vi "PRIME Detector Send START.vi"(5 "Observation":T1={"Priority"=0, "ID"="", "Observer"="", "Obj Name"="", "Obj Type"="", "RA and DEC String"={"RA"="HH:MM:SS.nnn", "DEC"="DEG:arcmin:arcsec.nn"}, "Filter Wheel 1"="", "Filter Wheel 2"="", "Integration Time"=0.0, "Observation Status"=enum."Error", "Offsets"={"RA"=0.0, "DEC"=0.0, "ROT"=0.0}, "Images"=0, "Dither Options"={"Dither"=enum."None", "Dither Radius"=0.0, "Dither Points"=0, "Dither Phase"=0.0}, "Comment 1"="", "Comment 2"=""}, 7 "Detector Config":T6={"Detector"=0, "Offsets"=[[0, 0, 0, 0, 0, 0, 0, 0, 0, 0, 0, 0, 0, 0, 0, 0, 0, 0, 0, 0, 0, 0, 0, 0, 0, 0, 0, 0, 0, 0, 0, 0]], "Detector Computer"={"Machine"="192.168.121.11", "Password"="rSL!nux23456", "FITS File Path"="", "Port"=44444, "Header Path"="", "Name"=""}, "FITS hdr template0"=path "", "FITS hdr template1"=path "", "FITS Data File Path"=path "", "FITS Detector Settings"={"Exp Time Short"=0.0, "# of Frames"=0.0, "Exp Time Long"=0.0, "# of Groups"=0.0, "Object Name"="", "Object"="", "Obs Type"="", "Image Type"="", "Observer"="", "Observer Affiliation"=""}, "Sim Folder"=path "", "Integration Mode"=enum."SSR", "Integration Time"=0.0, "Frame Int Time"=0.0} {"Offsets" format="%04x"; "Detector" items=["0", "1", "2"]}, 8 "error in (no error)":errorcluster, 9 "timeout (120s)":dbl=120.0, 10 "Exposure Time":dbl, 11 "connection ID":refnum<k5>[](array[refnum])) -> (0 "error out":errorcluster, 1 "Image Map":map{string, T10}(c390), 2 "Status out":T11, 3 "connection ID out":refnum<k5>[](array[refnum]))   [LabVIEW 2024, in "PRIME Detector.lvclass"]
uses:
  PRIME Detector.lvclass
  PRIME Detector cluster Status.ctl
  Detector Image typedef cluster.ctl
  RIMAS Detector Config.ctl
  RIMAS Detector Server Config.ctl
  RIMAS Observation Config.ctl
  Detector enum Detector Integration Mode.ctl
  typedefs/CC cluster Observation.ctl
  Observation Queue/CC enum Observation Status.ctl
  Telescope/CC cluster Telescope Offsets.ctl
  typedefs/CC cluster Observation Dither Options.ctl
  typedefs/CC enum Dither Selection.ctl
  3c100308-56f2-4219-aefe-58094781b1bc.vi
  Detector Class.lvclass
panel:
  out "Status":string
  out "Responses":string[](array[string])
  # "sec"
  # "sec"
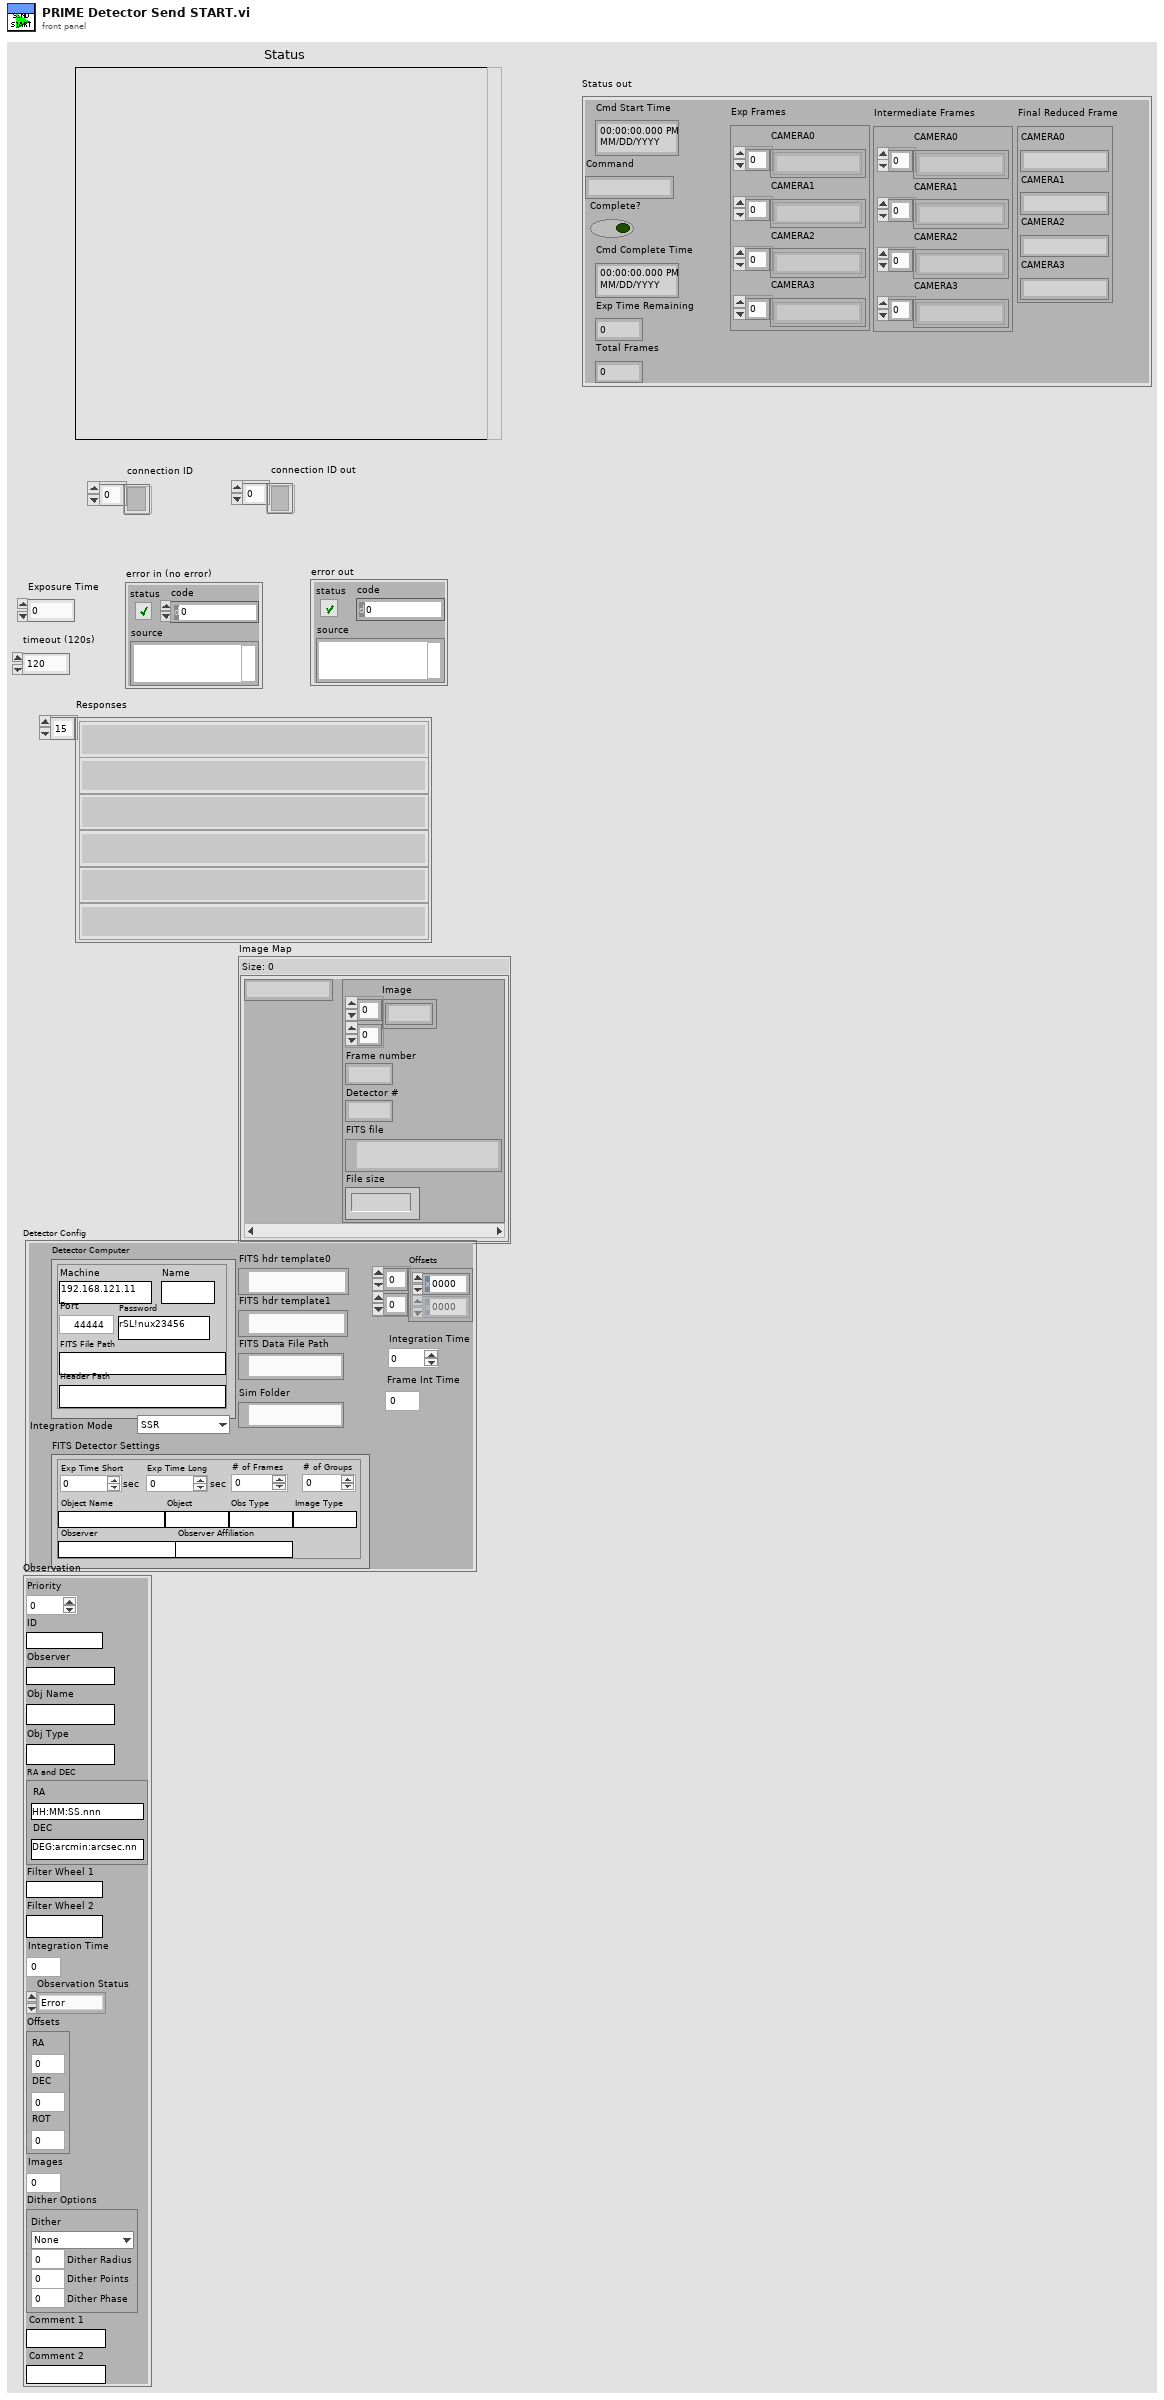
[diagram p1: front panel]
types:
  T1 = typedef "CC cluster Observation.ctl" = cluster{"Priority":i32, "ID":string, "Observer":string, "Obj Name":string, "Obj Type":string, "RA and DEC String":cluster{"RA":string, "DEC":string}, "Filter Wheel 1":string, "Filter Wheel 2":string, "Integration Time":dbl, "Observation Status":T2, "Offsets":T3, "Images":i32, "Dither Options":T4, "Comment 1":string, "Comment 2":string}
  T2 = typedef "CC enum Observation Status.ctl" = enum16{"Ready", "Running", "Done", "Error"}
  T3 = typedef "CC cluster Telescope Offsets.ctl" = cluster{"RA":dbl, "DEC":dbl, "ROT":dbl}
  T4 = typedef "CC cluster Observation Dither Options.ctl" = cluster{"Dither":T5, "Dither Radius":dbl, "Dither Points":i32, "Dither Phase":dbl}
  T5 = typedef "CC enum Dither Selection.ctl" = enum16{"None", "Circle", "Random"}
  T6 = typedef "RIMAS Detector Config.ctl" = cluster{"Detector":u16, "Offsets":u16[][], "Detector Computer":T7, "FITS hdr template0":path, "FITS hdr template1":path, "FITS Data File Path":path, "FITS Detector Settings":T8, "Sim Folder":path, "Integration Mode":T9, "Integration Time":dbl, "Frame Int Time":dbl}
  T7 = typedef "RIMAS Detector Server Config.ctl" = cluster{"Machine":string, "Password":string, "FITS File Path":string, "Port":u16, "Header Path":string, "Name":string}
  T8 = typedef "RIMAS Observation Config.ctl" = cluster{"Exp Time Short":dbl, "# of Frames":dbl, "Exp Time Long":dbl, "# of Groups":dbl, "Object Name":string, "Object":string, "Obs Type":string, "Image Type":string, "Observer":string, "Observer Affiliation":string}
  T9 = typedef "Detector enum Detector Integration Mode.ctl" = enum16{"SSR", "CDS", "MEAN", "MEDIAN", "MODE", "MIIN", "MAX"}
  T10 = typedef "Detector Class.lvclass/Detector Image typedef cluster.ctl" = cluster{"Image":sgl[][], "Frame number":i32, "Detector #":u16, "FITS file":path, "File size":i64}
  T11 = typedef "PRIME Detector cluster Status.ctl" = cluster{"Cmd Start Time":timestamp, "Command":string, "Complete?":bool, "Cmd Complete Time":timestamp, "Exp Time Remaining":dbl, "Total Frames":i32, "Exp Frames":cluster{"CAMERA0":string[], "CAMERA1":string[], "CAMERA2":string[], "CAMERA3":string[]}, "Intermediate Frames":cluster{"CAMERA0":string[], "CAMERA1":string[], "CAMERA2":string[], "CAMERA3":string[]}, "Final Reduced Frame":cluster{"CAMERA0":string, "CAMERA1":string, "CAMERA2":string, "CAMERA3":string}}
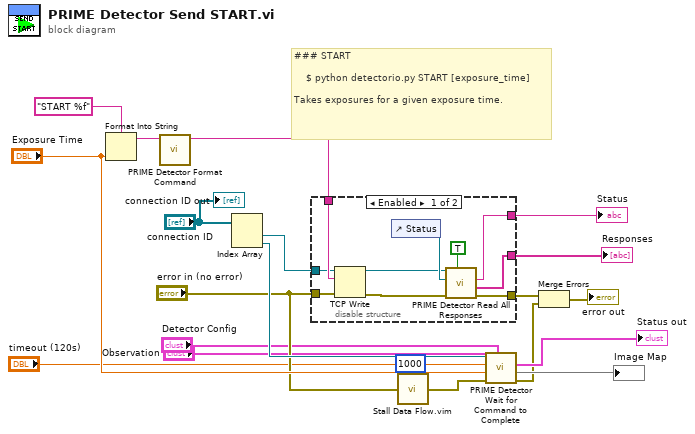
[diagram p0: block diagram]
diagram:
  # "### START\n\n    $ python detectorio.py START [exposure_time]\n\nTakes exposures for a given exposure time."
  n1 = Format Into String(format string="START %f" ("Command"), "Exposure Time") -> (resulting string=w14:string)  [unwired: 2 in, 1 out]
  n2 = call "PRIME Detector Format Command.vi"("Command"=w14) -> ("TCP String"=w20:string)  [unwired: 10 in]
  n3 = Index Array(array="connection ID") -> (element #1=w16:refnum<k5>, element #2=w13:refnum<k5>)  [unwired: 2 in]
  n4 = disable-structure shown="Enabled" {
    disable-tunnel: w20 -> [w30 _]
    disable-tunnel: "error in (no error)" -> [w29 _]
    disable-tunnel: [w28 _] -> w19
    disable-tunnel: [w27 _] -> w17
    disable-tunnel: w16 -> [w25 _]
    disable-tunnel: [w23 _] -> w15
    frame Enabled {
      n5 = TCP Write(connection ID=w25, data in=w30, error in (no error)=w29) -> (connection ID out=w24:refnum<k5>, error out=w21:errorcluster)  [unwired: 1 in, 1 out]
      n6 = control-ref of="Status"() -> (w26:refnum<vi>)
      n7 = call "PRIME Detector Read All Responses.vi"("Log"=TRUE, "error in"=w21, "Str Ref"=w26, "connection ID"=w24) -> ("error out"=w28:errorcluster, "Responses"=w27:string[], "Status Response"=w23:string)  [unwired: 4 in, 1 out]
    }
    frame Disabled {
    }
  }
  "Responses" <- w17
  "Status" <- w15
  n8 = call "Stall Data Flow.vim"("value in"="error in (no error)", "milliseconds to wait"=u32 1000) -> ("value out"=w7:errorcluster)  [unwired: 1 out]
  n9 = call "PRIME Detector Wait for Command to Complete.vi"("Observation"="Observation", "Detector Config"="Detector Config", "error in (no error)"=w7, "Exp Time"="Exposure Time", "timeout (120s)"="timeout (120s)", "connection ID"=w13) -> ("error out"=w8:errorcluster, "Image Map"=→"Image Map":map{string, T10}, "Status"=→"Status out":T11)  [unwired: 2 in, 1 out]
  n10 = Merge Errors(w19, w8) -> (→"error out":errorcluster)
  "connection ID out" <- "connection ID"
